vi "Wrapper.vi"(8 "error in (no error)":errorcluster, 10 "Actor in":refnum<class "Actor.lvclass">, 11 "Update Device Setpoint MSG in":refnum<class "Update Ctl Device Setpoint MSG.lvclass">) -> (0 "error out":errorcluster)   [LabVIEW 2017, in "Controller.lvlib" / "Update Ctl Device Setpoint MSG.lvclass"]
uses:
  Update Ctl Device Setpoint MSG.lvclass
  <vilib>/ActorFramework/Actor/Actor.lvclass
  gController.lvclass
  C:/Program Files (x86)/National Instruments/LabVIEW 2017/vi.lib/MSR Consulting, LLC/General Reuse/SuperActor/SuperActor.lvclass
  Update Ctl Device Setpoint MSG.lvclass/Update Ctl Device Setpoint MSG.ctl
  <vilib>/ActorFramework/Message Enqueuer/Message Enqueuer.lvclass
  Update Device Setpoint MSG/Update Device Setpoint MSG.lvclass
  C:/Program Files (x86)/National Instruments/LabVIEW 2017/vi.lib/ActorFramework/Message/Message.lvclass
  <vilib>/MSR Consulting, LLC/General Reuse/SuperActor/SuperActor.lvclass/SuperActor.ctl
  Update Device Setpoint MSG/Update Device Setpoint MSG.lvclass/Update Device Setpoint MSG.ctl
  <vilib>/ActorFramework/Message Enqueuer/Message Enqueuer.lvclass/Message Enqueuer.ctl
  Update Device Setpoint MSG/Write sp.vi
  <vilib>/MSR Consulting, LLC/General Reuse/SuperActor/Read EnqueuerMap.vi
  <vilib>/ActorFramework/Message Priority Queue/Priority Enqueue.vi
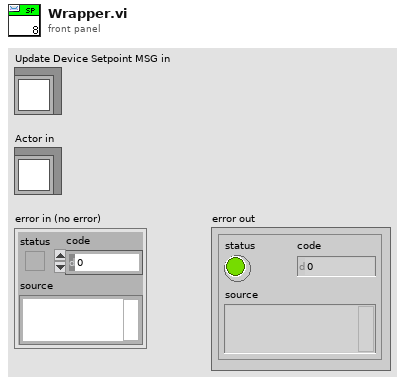
[diagram p1: front panel]
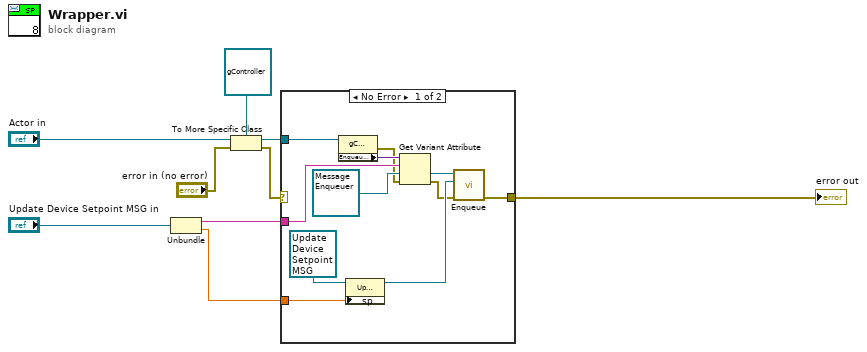
[diagram p0: block diagram]
diagram:
  n1 = Unbundle("Update Device Setpoint MSG in") -> (w5:string, w7:dbl)
  n2 = To More Specific Class(target class=refnum<class "gController.lvclass"> refnum ("Controller.lvlib:gController"), reference="Actor in", error in="error in (no error)") -> (specific class reference=w4:refnum<class "gController.lvclass">, error out=w6:errorcluster)
  n3 = case shown="No Error" w6 {
    selector: w6 -> [_ w21]
    tunnel: w4 -> [w20 _]
    tunnel: w5 -> [w17 _]
    tunnel: w7 -> [w13 _]
    tunnel: [w10 w21] -> w8
    frame No Error {
      n4 = property class="gController"(reference=w20) -> (error out=w16:errorcluster, "EnqueuerMap"=w19:variant)  [unwired: 1 in, 1 out]
      n5 = property class="Update Device Setpoint MSG.lvcl"(reference=refnum<class "Update Device Setpoint MSG.lvclass"> refnum ("DAQ Device.lvlib:Update Device Setpoint MSG.lvclass"), "sp"=w13) -> (reference out=w12:refnum<class "Update Device Setpoint MSG.lvclass">)  [unwired: 1 in, 1 out]
      n6 = Get Variant Attribute(Variant=w19, name=w17, default value (empty Variant)=refnum<class "Message Enqueuer.lvclass"> refnum ("Self Enqueuer"), error in=w16) -> (value=w15:refnum<class "Message Enqueuer.lvclass">, error out=w11:errorcluster)  [unwired: 2 out]
      n7 = call <vilib>:"Enqueue.vi"("error in (no error)"=w11, "Message"=w12, "Message Enqueuer in"=w15) -> ("error out"=w10:errorcluster)  [unwired: 7 in, 1 out]
    }
    frame Error {
    }
  }
  "error out" <- w8
